vi "Paser_Json_dev_to_cluster.vi"(8 "error in (no error)":errorcluster, 11 "USB_DEV_IN":string) -> (0 "error out":errorcluster, 1 "USB_DEV_OUT":string, 3 "DEV_BUSY":T1)   [LabVIEW 2015]
uses:
  Share Data/uPower_kit.ctl
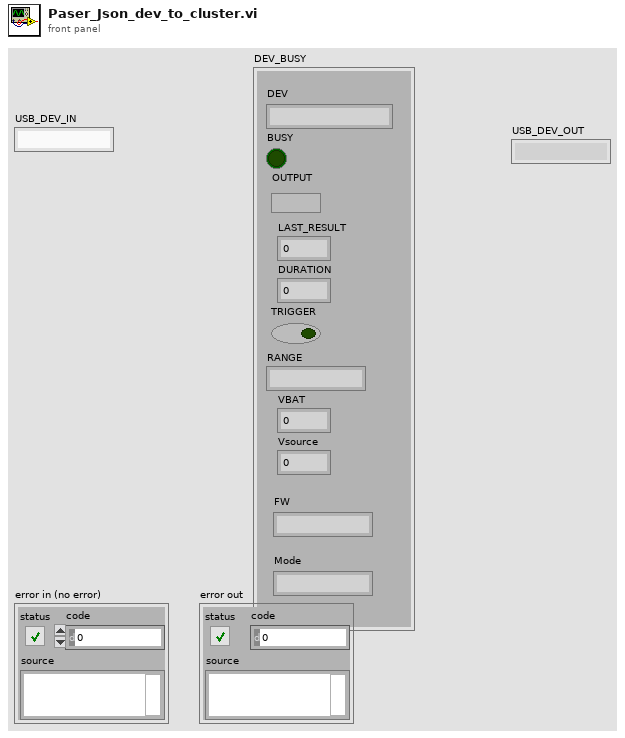
[diagram p1: front panel]
types:
  T1 = typedef "uPower_kit.ctl" = cluster{"DEV":string, "BUSY":bool, "VBAT":dbl, "OUTPUT":bool, "LAST_RESULT":dbl, "DURATION":u16, "TRIGGER":bool, "RANGE":string, "Vsource":dbl, "FW":string, "Mode":string}
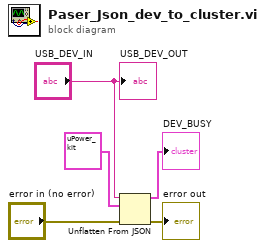
[diagram p0: block diagram]
diagram:
  n1 = Unflatten From JSON(JSON string="USB_DEV_IN", type and defaults=T1 {"DEV"="", "BUSY"=FALSE, "VBAT"=0.0, "OUTPUT"=FALSE, "LAST_RESULT"=0.0, "DURATION"=0, "TRIGGER"=FALSE, "RANGE"="", "Vsource"=0.0, "FW"="", "Mode"=""} ("DEV_BUSY"), error in (no error)="error in (no error)") -> (value=→"DEV_BUSY":T1, error out=→"error out":errorcluster)  [unwired: 4 in]
  "USB_DEV_OUT" <- "USB_DEV_IN"
